vi "FTW-Message-Request-WriteResponse.vi"(8 "error in":errorcluster, 9 "Response Body":string, 11 "FTW Incoming Request":refnum<class "FTW-Message-HttpRequest.lvclass">) -> (0 "error out":errorcluster, 3 "FTW Incoming Request out":refnum<class "FTW-Message-HttpRequest.lvclass">)   [LabVIEW 2015, in "FTW-Message-HttpRequest.lvclass"]
uses:
  FTW-Message-HttpRequest.lvclass
panel:
  # "Inputs"
  # "Outputs"
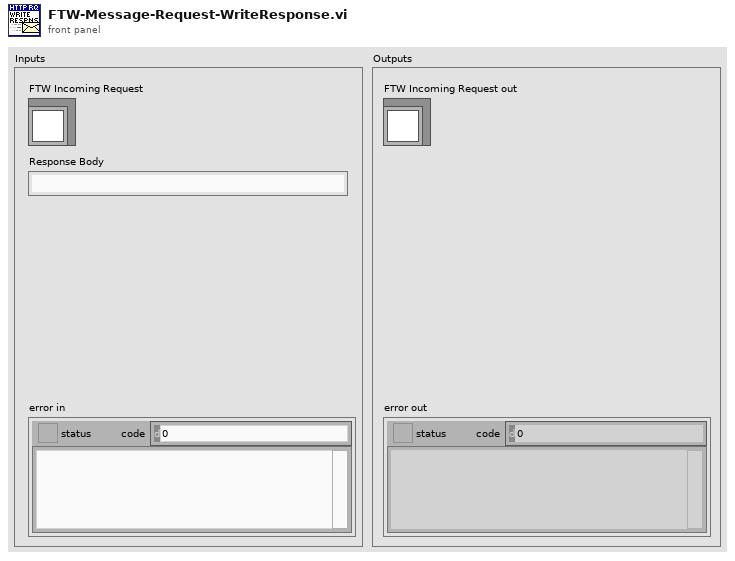
[diagram p1: front panel]
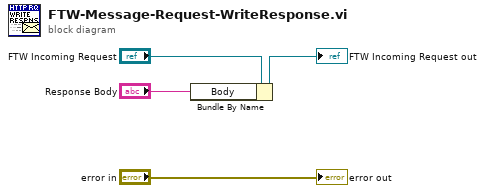
[diagram p0: block diagram]
diagram:
  n1 = Bundle By Name(cluster="FTW Incoming Request", "Body"="Response Body") -> (→"FTW Incoming Request out":refnum<class "FTW-Message-HttpRequest.lvclass">)
  "error out" <- "error in"
